vi "Tree_resync user event.vi"() -> (3 "Open/close":refnum<user-event>)   [LabVIEW 2023]
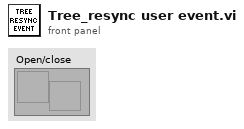
[diagram p1: front panel]
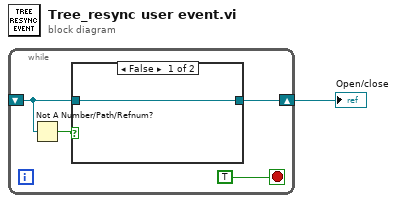
[diagram p0: block diagram]
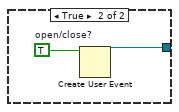
[diagram p2: hidden frame]
diagram:
  n1 = while {
    shift-right: [w5] -> w1
    shift-left: _ -> [w3]
    stop <- TRUE stop-if-true
    n2 = Not A Number/Path/Refnum?(number/path/refnum=w3) -> (NaN/Path/Refnum?=w4:bool)
    n3 = case shown="False" w4 {
      tunnel: [w6 w7] -> w5
      tunnel: w3 -> [w6 _]
      frame False {
      }
      frame True {
        w8 = TRUE  # open/close?
        n4 = Create User Event(user event datatype=w8) -> (user event=w7:refnum<user-event>)  [unwired: 1 in, 1 out]
      }
    }
  }
  "Open/close" <- w1
